vi "Control Motor.vi"(0 "Sines?":bool, 1 "Command":enum16{"Initialize", "Home", "Run", "Disable"}(ring), 2 "Re-center\nmotor":bool, 3 "DO Task":refnum<k21>="BlueSimple_DO", 5 "Sine parameters":T2={"Frequency"=0.5, "Degrees\npk-pk"=90.0, "Cycles"=10000} {"Degrees\npk-pk" min=0.1 max=120.0; "Frequency" min=0.001 format="%#_4g"}, 7 "Override bumps":bool, 9 "Home":bool, 11 "Bumps":bool, 12 "Bump timing":cluster{"Fix":dbl, "Rnd":dbl}={"Fix"=0.5, "Rnd"=0.5} {"Rnd" format="%.4f"; "Fix" format="%_4g"}, 13 "Start bump timer?":bool, 14 "Bump Parameters":T1={"Distance (deg)"=2.0, "Travel time (ms)"=500.0} {"Travel time (ms)" min=0.1 max=10000.0; "Distance (deg)" min=0.1}) -> (8 "Reset\nrecenter":bool, 10 "Reset override bumps":bool, 15 "Reset start button":bool)   [LabVIEW 2010]
panel:
  # "Motor"
  # "+"
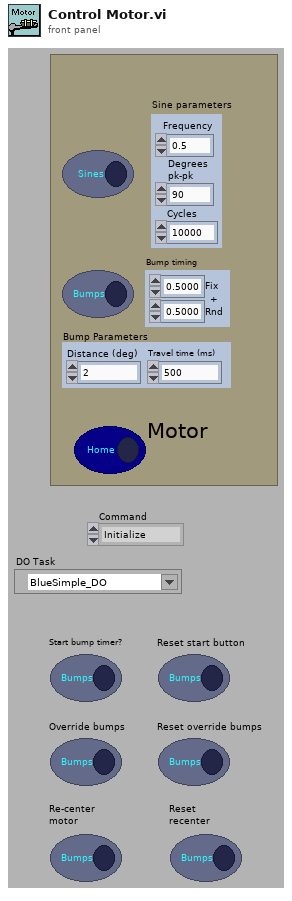
[diagram p1: front panel]
types:
  T1 = cluster{"Distance (deg)":dbl, "Travel time (ms)":dbl}
  T2 = cluster{"Frequency":dbl, "Degrees\npk-pk":dbl, "Cycles":i16}
  T3 = cluster{"Sines?":bool, "Sine parameters":cluster{"Frequency":dbl, "Degrees\npk-pk":dbl, "Cycles":i16}}
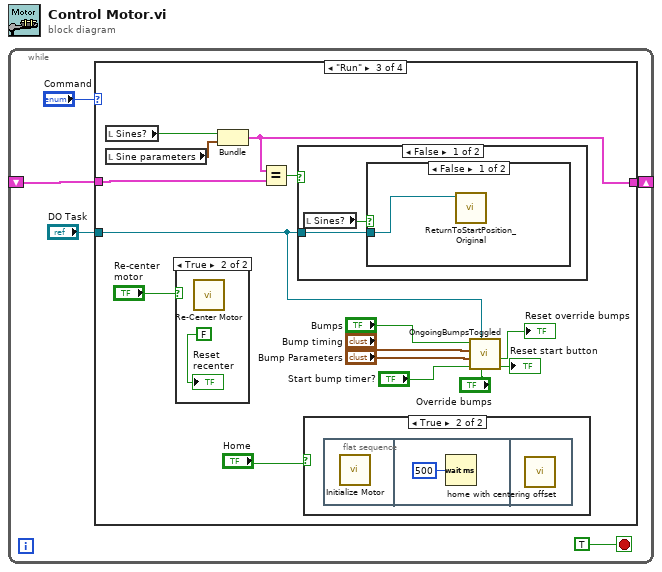
[diagram p0: block diagram]
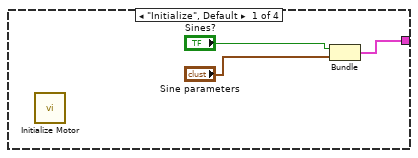
[diagram p2: hidden frame]
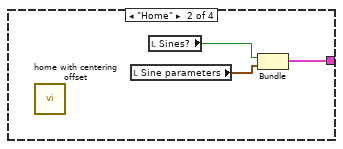
[diagram p3: hidden frame]
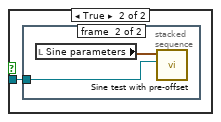
[diagram p6: hidden frame]
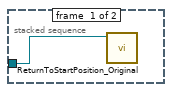
[diagram p7: hidden frame]
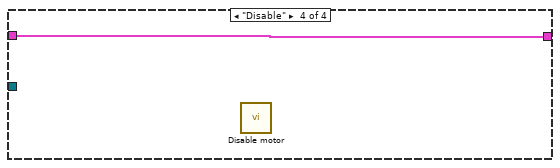
[diagram p9: hidden frame]
diagram:
  n1 = while {
    shift-right: [w4] -> _
    shift-left: _ -> [w3]
    stop <- TRUE stop-if-true
    n2 = case shown="\"Run\"" "Command" {
      tunnel: [w6 w9 w23 w36] -> w4
      tunnel: w3 -> [_ _ w24 w36]
      tunnel: "DO Task" -> [_ _ w12 _]
      frame "Initialize", Default {
        n3 = call "Initialize Motor.vi"() -> ()  [unwired: 1 in]
        n4 = Bundle("Sines?"="Sines?", "Sine parameters"="Sine parameters") -> (w6:T3)  [unwired: 1 in]
      }
      frame "Home" {
        n5 = call "home with centering offset.vi"() -> ()  [unwired: 1 in]
        n6 = local read "Sine parameters"() -> (w10:T2)
        n7 = local read "Sines?"() -> (w11:bool)
        n8 = Bundle("Sines?"=w11, "Sine parameters"=w10) -> (w9:T3)  [unwired: 1 in]
      }
      frame "Run" {
        n9 = local read "Sines?"() -> (w26:bool)
        n10 = local read "Sine parameters"() -> (w25:T2)
        n11 = case shown="True" "Re-center\nmotor" {
          frame False {
          }
          frame True {
            n12 = call "Re-Center Motor.vi"() -> ()  [unwired: 8 in, 2 out]
            "Reset\nrecenter" <- FALSE ("Reset\nrecenter")
          }
        }
        n13 = Bundle("Sines?"=w26, "Sine parameters"=w25) -> (w23:T3)  [unwired: 1 in]
        n14 = Equal?(x=w23, y=w24) -> (x = y?=w22:bool)
        n15 = case shown="False" w22 {
          tunnel: w12 -> [w29 _]
          frame False {
            n16 = local read "Sines?"() -> (w30:bool)
            n17 = case shown="False" w30 {
              tunnel: w29 -> [w31 w32]
              frame False {
                n18 = call "ReturnToStartPosition_Original.vi"("DO Task"=w31) -> ()  [unwired: 9 in]
              }
              frame True {
                n19 = stacked-sequence {
                  tunnel: w32 -> [w33 w34]
                  frame #0 {
                    n20 = call "ReturnToStartPosition_Original.vi"("DO Task"=w33) -> ()  [unwired: 9 in]
                  }
                  frame #1 {
                    n21 = local read "Sine parameters"() -> (w35:T2)
                    n22 = call "Sine test with pre-offset.vi"("DO Task"=w34, "Sine parameters"=w35) -> ()  [unwired: 3 in, 1 out]
                  }
                }
              }
            }
          }
          frame True {
          }
        }
        n23 = case shown="True" "Home" {
          frame False {
          }
          frame True {
            n24 = flat-sequence {
              frame #0 {
                n25 = call "Initialize Motor.vi"() -> ()  [unwired: 1 in]
              }
              frame #1 {
                n26 = Wait (ms)(milliseconds to wait=u32 500) -> ()  [unwired: 1 out]
              }
              frame #2 {
                n27 = call "home with centering offset.vi"() -> ()  [unwired: 1 in]
              }
            }
          }
        }
        n28 = call "OngoingBumpsToggled.vi"("Override bumps"="Override bumps", "DO Task"=w12, "Start \nbump timer?"="Start bump timer?", "Bump Parameters"="Bump Parameters", "Bump timing"="Bump timing", "Bumps on?"="Bumps") -> ("Reset start button"=→"Reset start button":bool, "Reset override bumps"=→"Reset override bumps":bool)  [unwired: 4 in]
      }
      frame "Disable" {
        n29 = call "Disable motor.vi"() -> ()  [unwired: 1 in]
      }
    }
  }
